vi "updateStiffnessLog.vi"(8 "error in (no error)":errorcluster, 11 "Model in":refnum<class "Model.lvclass">) -> (0 "error out":errorcluster, 3 "Model out":refnum<class "Model.lvclass">)   [LabVIEW 2013]
uses:
  <userlib>/Common/Log/Log/Log.lvclass
  Model.lvclass
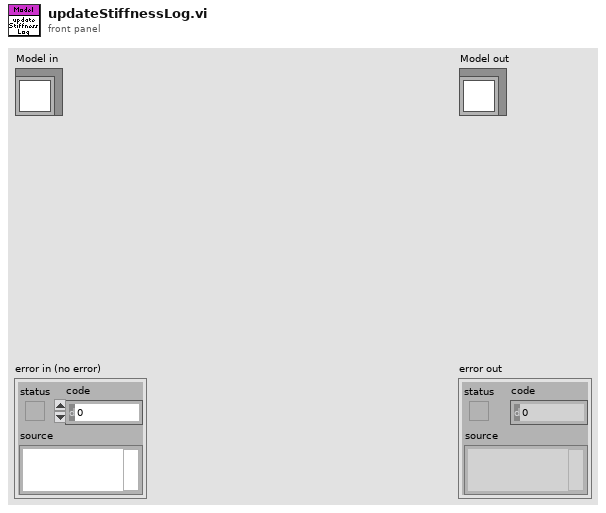
[diagram p1: front panel]
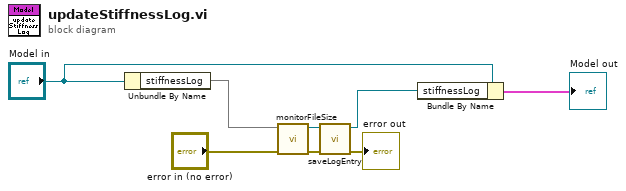
[diagram p0: block diagram]
diagram:
  n1 = Unbundle By Name("Model in") -> ("stiffnessLog"=w6)
  n2 = call <userlib>:"monitorFileSize.vi"("error in (no error)"="error in (no error)", "Logger in"=w6) -> ("error out"=w8:errorcluster, "Logger out"=w7:refnum<class "Log.lvclass">)  [unwired: 6 in, 2 out]
  n3 = call-dynamic "saveLogEntry.vi"("error in (no error)"=w8, "Logger in"=w7) -> ("error out"=→"error out":errorcluster, "Logger out"=w4:refnum<class "Log.lvclass">)  [unwired: 8 in]
  n4 = Bundle By Name(cluster="Model in", "stiffnessLog"=w4) -> (→"Model out":cluster{})
